vi "API_Example.vi"(0 "DLP2 in":refnum<class "DLP2.lvclass">, 1 "Wait (F)":bool, 5 "Table":string, 7 "InventoryRecord.Stocker":T1 items=["Main", "Exp1", "Exp2"], 11 "error in (no error)":errorcluster, 12 "Timeout (ms)":u32) -> (4 "DLP2 out":refnum<class "DLP2.lvclass">, 6 "Slot":string, 15 "error out":errorcluster)   [LabVIEW 2022 SP3, in "DLP2.lvclass"]
doc: "Developed by Kevin Thompson\nkevin@thompsonengineering.net\n\nCopyright 2018\nThompson Engineering, LLC"
uses:
  DLP2.lvclass
  DLP2.lvclass/DLP2.ctl
  DataTypes/AsynCmd_Temp01--enum.ctl
  Database/DataTypes/SQLQuery--Enum.ctl
  Database/DataTypes/GenericQuery--Cluster.ctl
  Database/DataTypes/Stocker--Enum.ctl
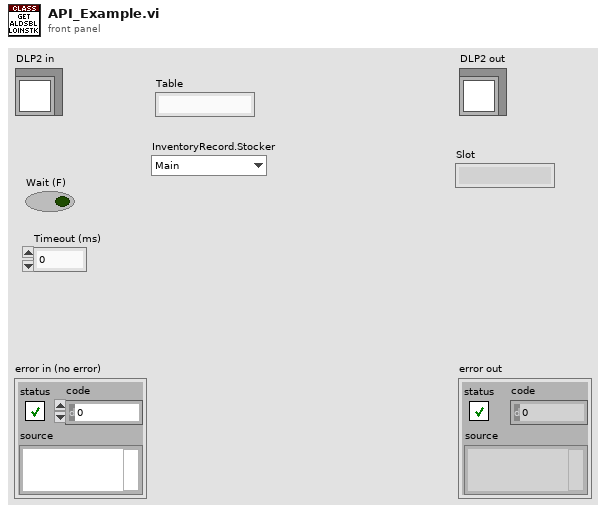
[diagram p1: front panel]
types:
  T1 = typedef "Stocker--Enum.ctl" = u16
  T2 = typedef "SQLQuery--Enum.ctl" = enum16{"GetAllMaterials", "GetAllColors"}
  T3 = typedef "GenericQuery--Cluster.ctl" = cluster{"Query":T2, "Table":string}
  T4 = typedef "DLP2.lvclass/AsynCmd_Temp01--enum.ctl" = enum16{"DB.DeleteRecord", "DB.UpdateRecord", "DB.InsertRecord", "DB.SelectRecord", "DB.ExecuteSQLCommand", "DB.FindFirstSlot", "DB.GenericSQLQuery"}
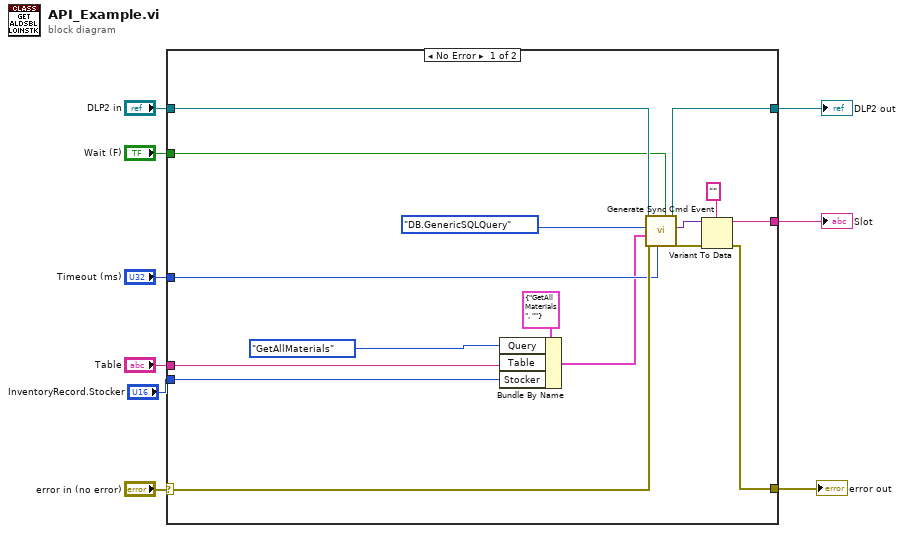
[diagram p0: block diagram]
diagram:
  n1 = case shown="No Error" "error in (no error)" {
    selector: "error in (no error)" -> [w23 w27]
    tunnel: [w18 w27] -> w8
    tunnel: [w24 w26] -> w6
    tunnel: "DLP2 in" -> [w25 w26]
    tunnel: [w20 _] -> w3
    tunnel: "Wait (F)" -> [w17 _]
    tunnel: "Timeout (ms)" -> [w16 _]
    tunnel: "Table" -> [w11 _]
    tunnel: "InventoryRecord.Stocker" -> [w10 _]
    frame No Error {
      n2 = Bundle By Name(cluster=T3 {"Query"=enum."GetAllMaterials", "Table"=""}, "Query"=SQLQuery--Enum."GetAllMaterials", "Table"=w11, "Stocker"=w10) -> (w12:T3)
      n3 = call "Generate Sync Cmd Event.vi"("Wait (F)"=w17, "Timeout (ms)"=w16, "error in (no error)"=w23, "vData"=w12, "AsyncCmd"=AsynCmd_Temp01--enum."DB.GenericSQLQuery", "DLP2 in"=w25) -> ("error out"=w19:errorcluster, "Return Value"=w21:variant, "DLP2 out"=w24:refnum<class "DLP2.lvclass">)  [unwired: 3 in]
      n4 = Variant To Data(error in=w19, type="", Variant=w21) -> (data=w20:string, error out=w18:errorcluster)
    }
    frame Error {
    }
  }
  "error out" <- w8
  "DLP2 out" <- w6
  "Slot" <- w3
